vi "Send Toggle Output.vi"(8 "error in":errorcluster, 11 "69X_79X in":refnum<class "69X_79X.lvclass">) -> (0 "error out":errorcluster, 3 "69X_79X out":refnum<class "69X_79X.lvclass">)   [LabVIEW 2019, in "69X_79X.lvlib" / "69X_79X.lvclass"]
uses:
  Library/69X_79X.lvclass
  C:/Users/Public/Documents/Development/builds/Instruments/PowerSupply.lvlibp/Library/PowerSupply.lvclass
  Accessors/Read Local Resource.vi
  Accessors/Write Local Resource.vi
  <instrlib>/Agilent N6900 N7900 Series/Agilent N6900 N7900 Series.lvlib
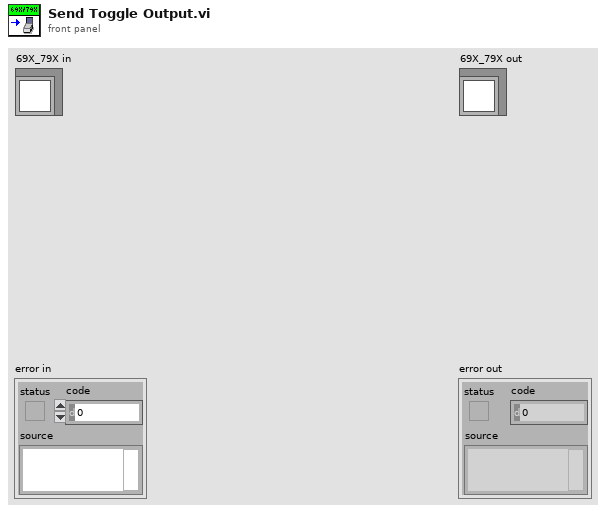
[diagram p1: front panel]
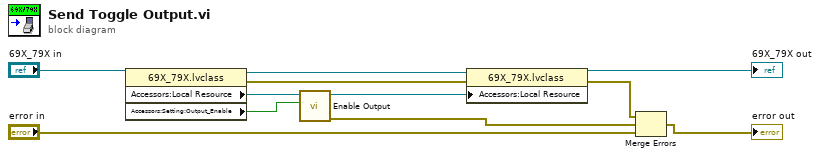
[diagram p0: block diagram]
diagram:
  n1 = property class="69X_79X.lvclass"(reference="69X_79X in") -> (reference out=w8:refnum<class "69X_79X.lvclass">, error out=w7:errorcluster, "Accessors:Local Resource"=w10:refnum<visa-resource-name>, "Accessors:Setting:Output_Enable"=w9:bool)  [unwired: 1 in]
  n2 = call <instrlib>:"Enable Output.vi"("Enable Output (F: Disable)"=w9, "VISA resource name"=w10) -> ("error out"=w4:errorcluster, "VISA resource name out"=w3:refnum<visa-resource-name>)  [unwired: 8 in]
  n3 = property class="69X_79X.lvclass"(reference=w8, error in=w7, "Accessors:Local Resource"=w3) -> (reference out=→"69X_79X out":refnum<class "69X_79X.lvclass">, error out=w5:errorcluster)
  n4 = Merge Errors(w5, w4, "error in") -> (→"error out":errorcluster)
